vi "Abadines_Server3.vi"() -> ()   [LabVIEW 2013]
uses:
  <vilib>/NXT/Block Support/NXT_InputPort.ctl
  <vilib>/NXT/Block Support/NXT_MessageMailbox.ctl
  <vilib>/NXT/Block Support/NXT_OutputPort.ctl
  <vilib>/NXT/Subs/MotorOutput.ctl
  <vilib>/NXT/Dual Mode Library/BT/BlueTooth_Write_Num.vi
  <vilib>/NXT/NXTIO Xnodes/NXTIONodeSubVIs/NXTStopMotors.vi
  <vilib>/NXT/Dual Mode Library/Display/drawNumber.vi
  <vilib>/NXT/NXTIO Xnodes/AddressXNode/NXTIOAddress.xnode
  <vilib>/NXT/NXTIO Xnodes/NXTIOXNode/NXTIO.xnode
  <vilib>/NXT/Subs/LVHSConnector.ctl
  <vilib>/NXT/LegoClasses/BrickReference/BrickReference.lvclass
  <vilib>/NXT/Dual Mode Library/Display/drawNumber_float.vi
panel:
  out "Case Accord. BJr.":i32
  out "Blue Line":i16
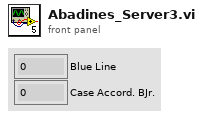
[diagram p1: front panel]
types:
  T1 = typedef "NXT_MessageMailbox.ctl" = u8
  T2 = typedef "LVHSConnector.ctl" = refnum<class "BrickReference.lvclass">
  T3 = typedef "NXT_OutputPort.ctl" = u8
  T4 = typedef "NXT_InputPort.ctl" = u32
  T5 = typedef "MotorOutput.ctl" = u8
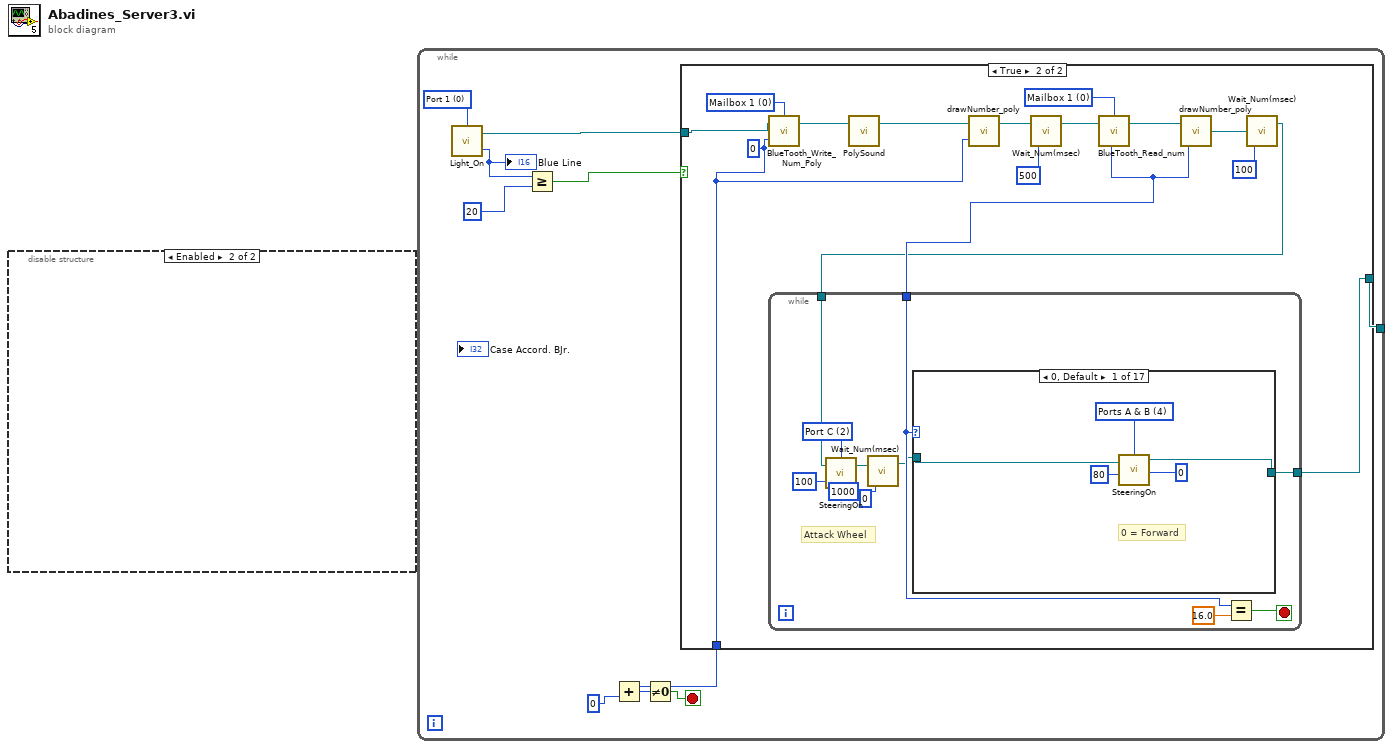
[diagram p0: block diagram]
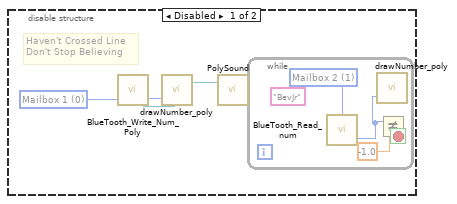
[diagram p2: hidden frame]
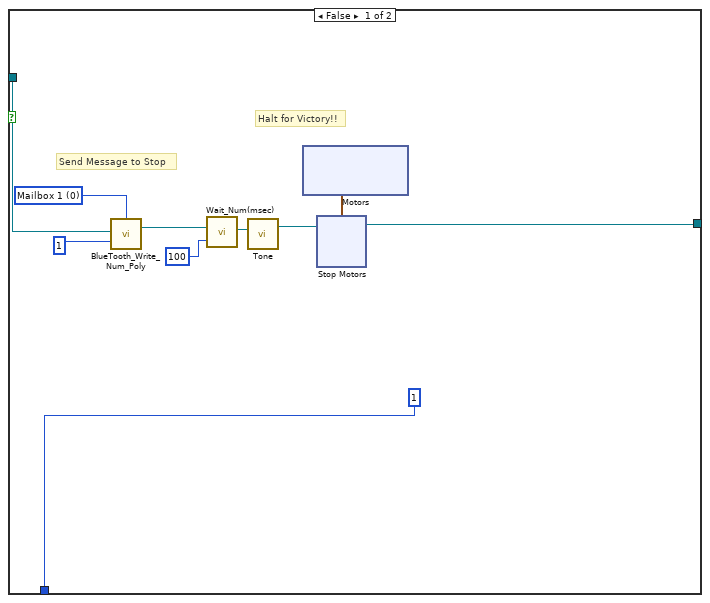
[diagram p3: hidden frame]
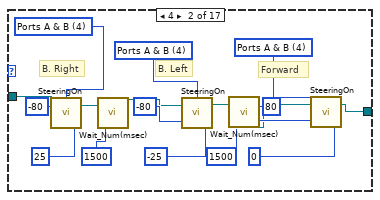
[diagram p4: hidden frame]
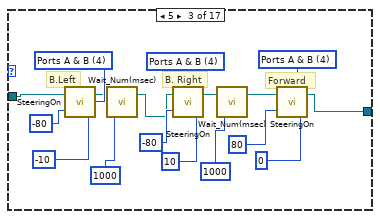
[diagram p5: hidden frame]
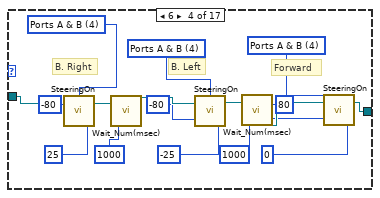
[diagram p6: hidden frame]
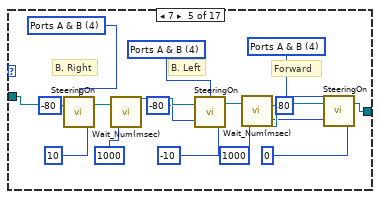
[diagram p7: hidden frame]
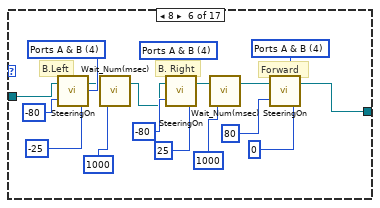
[diagram p8: hidden frame]
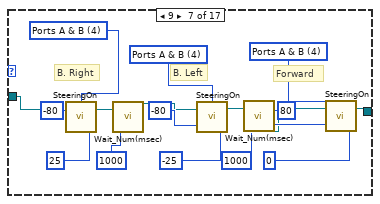
[diagram p9: hidden frame]
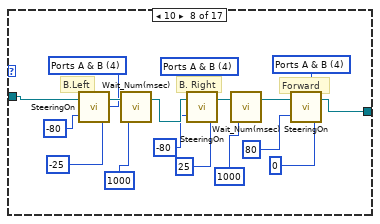
[diagram p10: hidden frame]
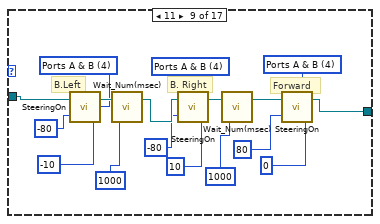
[diagram p11: hidden frame]
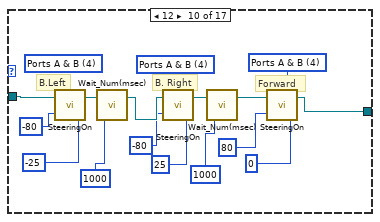
[diagram p12: hidden frame]
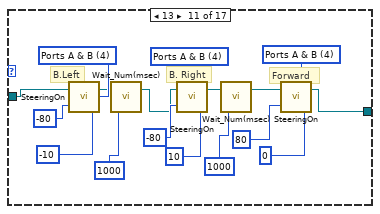
[diagram p13: hidden frame]
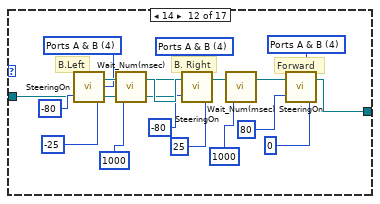
[diagram p14: hidden frame]
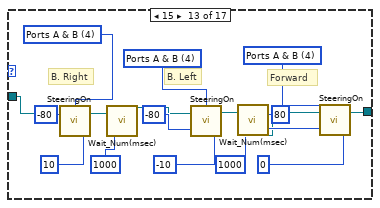
[diagram p15: hidden frame]
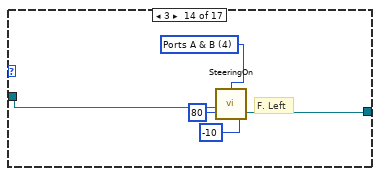
[diagram p16: hidden frame]
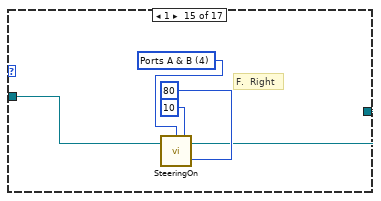
[diagram p17: hidden frame]
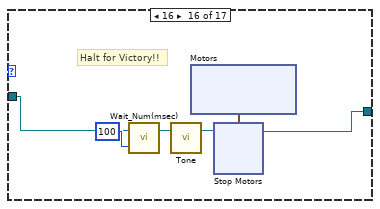
[diagram p18: hidden frame]
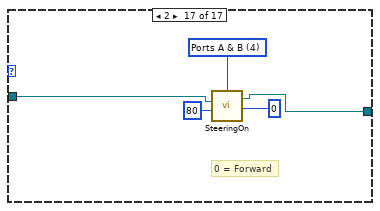
[diagram p19: hidden frame]
diagram:
  n1 = disable-structure shown="Enabled" {
    frame Disabled {
      w1 = T1 0 items=["Mailbox 1", "Mailbox 2", "Mailbox 3", "Mailbox 4", "Mailbox 5", "Mailbox 6", "Mailbox 7", "Mailbox 8", "Mailbox 9", "Mailbox 10"] ("Mailbox")
      # "Haven't Crossed Line\nDon't Stop Believing"
      n2 = call-poly <vilib>:"BlueTooth_Write_Num_Poly.vi"("Mailbox"=w1) -> ("Message"=w4:i32, 2:"NXT/EV3"=w2:T2, 4:"NXT/EV3"=w3:T2)  [unwired: 1 in]
      n3 = call-poly <vilib>:"drawNumber_poly.vi"("number"=w4, "NXT/EV3"=w3) -> ()  [unwired: 2 in, 1 out]
      n4 = call-poly <vilib>:"PolySound.vi"("NXT/EV3"=w3) -> ()  [unwired: 3 in, 1 out]
      n5 = while {
        stop <- _ stop-if-true
        w9 = T1 1 items=["Mailbox 1", "Mailbox 2", "Mailbox 3", "Mailbox 4", "Mailbox 5", "Mailbox 6", "Mailbox 7", "Mailbox 8", "Mailbox 9", "Mailbox 10"] ("Mailbox")
        (unwired) "BevJr" ("Partner Name")
        n6 = call <vilib>:"BlueTooth_Read_num.vi"("Mailbox"=w9) -> ("Message"=w5:i32, 2:"NXT/EV3"=w8:T2, 4:"NXT/EV3"=w7:T2)  [unwired: 1 in]
        n7 = call-poly <vilib>:"drawNumber_poly.vi"("number"=w5) -> ()  [unwired: 3 in, 1 out]
        n8 = Not Equal?(x=w5, y=-1.0) -> ()  [unwired: 1 out]
      }
    }
    frame Enabled {
    }
  }
  n9 = while {
    tunnel: [w15] -> _
    stop <- w11 stop-if-true
    w19 = T4 0 items=["Port 1", "Port 2", "Port 3", "Port 4"] ("Port (Port 3)")
    n10 = call <vilib>:"Light_On.vi"("Port (Port 3)"=w19) -> ("Scaled Value"=w18:i16, "NXT/EV3"=w10:T2)  [unwired: 2 in]
    "Blue Line" <- w18
    n11 = Greater Or Equal?(x=w18, y=i16 20) -> (x >= y?=w16:bool)
    n12 = case shown="True" w16 {
      tunnel: w10 -> [w27 w40]
      tunnel: [w21 w38] -> w15
      tunnel: [1 w39] -> w14
      frame False {
        w28 = T1 0 items=["Mailbox 1", "Mailbox 2", "Mailbox 3", "Mailbox 4", "Mailbox 5", "Mailbox 6", "Mailbox 7", "Mailbox 8", "Mailbox 9", "Mailbox 10"] ("Mailbox")
        # "Halt for Victory!!"
        # "Send Message to Stop"
        n13 = call-poly <vilib>:"BlueTooth_Write_Num_Poly.vi"("Message"=1, "NXT/EV3"=w27, "Mailbox"=w28) -> ("NXT/EV3"=w23:T2)  [unwired: 1 in]
        n14 = call <vilib>:"Wait_Num(msec).vi"("Time (100 msec)"=u32 100, "NXT/EV3"=w23) -> ("NXT/EV3"=w24:T2)  [unwired: 2 in]
        n15 = call <vilib>:"Tone.vi"("NXT/EV3"=w24) -> ("NXT/EV3"=w22:T2)  [unwired: 3 in]
        n16 = xnode "Motors"() -> ("Motor"=w20:cluster{"Port":T3, "Port":T3})
        n17 = xnode "Stop Motors"("Motors"=w20, "NXT/EV3"=w22) -> ("NXT/EV3"=w21:T2)
      }
      frame True {
        w50 = T1 0 items=["Mailbox 1", "Mailbox 2", "Mailbox 3", "Mailbox 4", "Mailbox 5", "Mailbox 6", "Mailbox 7", "Mailbox 8", "Mailbox 9", "Mailbox 10"] ("Mailbox")
        w39 = 0 ("Message")
        w41 = T1 0 items=["Mailbox 1", "Mailbox 2", "Mailbox 3", "Mailbox 4", "Mailbox 5", "Mailbox 6", "Mailbox 7", "Mailbox 8", "Mailbox 9", "Mailbox 10"] ("Mailbox")
        n18 = call-poly <vilib>:"BlueTooth_Write_Num_Poly.vi"("Message"=w39, "NXT/EV3"=w40, "Mailbox"=w41) -> ("NXT/EV3"=w42:T2)  [unwired: 1 in]
        n19 = call-poly <vilib>:"PolySound.vi"("NXT/EV3"=w42) -> ("NXT/EV3"=w47:T2)  [unwired: 3 in]
        n20 = call-poly <vilib>:"drawNumber_poly.vi"("number"=w39, "NXT/EV3"=w47) -> ("NXT/EV3"=w44:T2)  [unwired: 2 in]
        n21 = call <vilib>:"Wait_Num(msec).vi"("Time (100 msec)"=u32 500, "NXT/EV3"=w44) -> ("NXT/EV3"=w45:T2)  [unwired: 2 in]
        n22 = call <vilib>:"BlueTooth_Read_num.vi"("NXT/EV3"=w45, "Mailbox"=w50) -> ("Message"=w37:i32, "NXT/EV3"=w43:T2)  [unwired: 1 in]
        n23 = call-poly <vilib>:"drawNumber_poly.vi"("number"=w37, "NXT/EV3"=w43) -> ("NXT/EV3"=w49:T2)  [unwired: 2 in]
        n24 = call <vilib>:"Wait_Num(msec).vi"("Time (100 msec)"=u32 100, "NXT/EV3"=w49) -> ("NXT/EV3"=w36:T2)  [unwired: 2 in]
        n25 = while {
          tunnel: [w61] -> w38
          tunnel: w37 -> [w54]
          tunnel: w36 -> [w60]
          stop <- w56 stop-if-true
          w59 = T5 2 items=["Port A"=0, "Port B"=1, "Port C"=2, "Ports A & B"=4, "Ports A & C"=5, "Ports B & C"=6, "All Ports"=3] ("Output Ports (A & B)")
          # "Attack Wheel"
          n26 = call <vilib>:"SteeringOn.vi"("Power (75)"=100, "Steering (100)"=0, "NXT/EV3"=w60, "Output Ports (A & B)"=w59) -> ("NXT/EV3"=w53:T2)
          n27 = call <vilib>:"Wait_Num(msec).vi"("Time (100 msec)"=u32 1000, "NXT/EV3"=w53) -> ("NXT/EV3"=w52:T2)  [unwired: 2 in]
          n28 = case shown="0, Default" w54 {
            tunnel: w52 -> [w64 w77 w85 w102 w119 w145 w153 w170 w187 w204 w220 w237 w255 w272 w277 w282 w294]
            tunnel: [w63 w76 w84 w101 w118 w144 w152 w169 w186 w203 w219 w236 w254 w271 w276 w283 w293] -> w61
            frame 0, Default {
              w62 = T5 4 items=["Port A"=0, "Port B"=1, "Port C"=2, "Ports A & B"=4, "Ports A & C"=5, "Ports B & C"=6, "All Ports"=3] ("Output Ports (A & B) 5")
              # "0 = Forward"
              n29 = call <vilib>:"SteeringOn.vi"("Power (75)"=80, "Steering (100)"=0, "NXT/EV3"=w64, "Output Ports (A & B)"=w62) -> ("NXT/EV3"=w63:T2)
            }
            frame 4 {
              w73 = T5 4 items=["Port A"=0, "Port B"=1, "Port C"=2, "Ports A & B"=4, "Ports A & C"=5, "Ports B & C"=6, "All Ports"=3] ("Output Ports (A & B) 15")
              w74 = T5 4 items=["Port A"=0, "Port B"=1, "Port C"=2, "Ports A & B"=4, "Ports A & C"=5, "Ports B & C"=6, "All Ports"=3] ("Output Port (All Ports) 6")
              w75 = T5 4 items=["Port A"=0, "Port B"=1, "Port C"=2, "Ports A & B"=4, "Ports A & C"=5, "Ports B & C"=6, "All Ports"=3] ("Output Ports (A & B) 16")
              # "Forward"
              # "B. Left"
              # "B. Right"
              n30 = call <vilib>:"SteeringOn.vi"("Power (75)"=-80, "Steering (100)"=25, "NXT/EV3"=w77, "Output Ports (A & B)"=w75) -> ("NXT/EV3"=w72:T2)
              n31 = call <vilib>:"Wait_Num(msec).vi"("Time (100 msec)"=u32 1500, "NXT/EV3"=w72) -> ("NXT/EV3"=w71:T2)  [unwired: 2 in]
              n32 = call <vilib>:"SteeringOn.vi"("Power (75)"=-80, "Steering (100)"=-25, "NXT/EV3"=w71, "Output Ports (A & B)"=w74) -> ("NXT/EV3"=w70:T2)
              n33 = call <vilib>:"Wait_Num(msec).vi"("Time (100 msec)"=u32 1500, "NXT/EV3"=w70) -> ("NXT/EV3"=w69:T2)  [unwired: 2 in]
              n34 = call <vilib>:"SteeringOn.vi"("Power (75)"=80, "Steering (100)"=0, "NXT/EV3"=w69, "Output Ports (A & B)"=w73) -> ("NXT/EV3"=w76:T2)
            }
            frame 5 {
              w92 = T5 4 items=["Port A"=0, "Port B"=1, "Port C"=2, "Ports A & B"=4, "Ports A & C"=5, "Ports B & C"=6, "All Ports"=3] ("Output Ports (A & B) 21")
              w93 = T5 4 items=["Port A"=0, "Port B"=1, "Port C"=2, "Ports A & B"=4, "Ports A & C"=5, "Ports B & C"=6, "All Ports"=3] ("Output Port (All Ports) 9")
              w94 = T5 4 items=["Port A"=0, "Port B"=1, "Port C"=2, "Ports A & B"=4, "Ports A & C"=5, "Ports B & C"=6, "All Ports"=3] ("Output Ports (A & B) 22")
              # "Forward"
              # "B. Right"
              # "B.Left"
              n35 = call <vilib>:"SteeringOn.vi"("Power (75)"=-80, "Steering (100)"=-10, "NXT/EV3"=w85, "Output Ports (A & B)"=w94) -> ("NXT/EV3"=w90:T2)
              n36 = call <vilib>:"Wait_Num(msec).vi"("Time (100 msec)"=u32 1000, "NXT/EV3"=w90) -> ("NXT/EV3"=w89:T2)  [unwired: 2 in]
              n37 = call <vilib>:"SteeringOn.vi"("Power (75)"=-80, "Steering (100)"=10, "NXT/EV3"=w89, "Output Ports (A & B)"=w93) -> ("NXT/EV3"=w87:T2)
              n38 = call <vilib>:"Wait_Num(msec).vi"("Time (100 msec)"=u32 1000, "NXT/EV3"=w87) -> ("NXT/EV3"=w86:T2)  [unwired: 2 in]
              n39 = call <vilib>:"SteeringOn.vi"("Power (75)"=80, "Steering (100)"=0, "NXT/EV3"=w86, "Output Ports (A & B)"=w92) -> ("NXT/EV3"=w84:T2)
            }
            frame 6 {
              w111 = T5 4 items=["Port A"=0, "Port B"=1, "Port C"=2, "Ports A & B"=4, "Ports A & C"=5, "Ports B & C"=6, "All Ports"=3] ("Output Ports (A & B) 15")
              w110 = T5 4 items=["Port A"=0, "Port B"=1, "Port C"=2, "Ports A & B"=4, "Ports A & C"=5, "Ports B & C"=6, "All Ports"=3] ("Output Port (All Ports) 6")
              w109 = T5 4 items=["Port A"=0, "Port B"=1, "Port C"=2, "Ports A & B"=4, "Ports A & C"=5, "Ports B & C"=6, "All Ports"=3] ("Output Ports (A & B) 16")
              # "Forward"
              # "B. Left"
              # "B. Right"
              n40 = call <vilib>:"SteeringOn.vi"("Power (75)"=-80, "Steering (100)"=25, "NXT/EV3"=w102, "Output Ports (A & B)"=w109) -> ("NXT/EV3"=w112:T2)
              n41 = call <vilib>:"Wait_Num(msec).vi"("Time (100 msec)"=u32 1000, "NXT/EV3"=w112) -> ("NXT/EV3"=w113:T2)  [unwired: 2 in]
              n42 = call <vilib>:"SteeringOn.vi"("Power (75)"=-80, "Steering (100)"=-25, "NXT/EV3"=w113, "Output Ports (A & B)"=w110) -> ("NXT/EV3"=w114:T2)
              n43 = call <vilib>:"Wait_Num(msec).vi"("Time (100 msec)"=u32 1000, "NXT/EV3"=w114) -> ("NXT/EV3"=w115:T2)  [unwired: 2 in]
              n44 = call <vilib>:"SteeringOn.vi"("Power (75)"=80, "Steering (100)"=0, "NXT/EV3"=w115, "Output Ports (A & B)"=w111) -> ("NXT/EV3"=w101:T2)
            }
            frame 7 {
              w128 = T5 4 items=["Port A"=0, "Port B"=1, "Port C"=2, "Ports A & B"=4, "Ports A & C"=5, "Ports B & C"=6, "All Ports"=3] ("Output Ports (A & B) 15")
              w127 = T5 4 items=["Port A"=0, "Port B"=1, "Port C"=2, "Ports A & B"=4, "Ports A & C"=5, "Ports B & C"=6, "All Ports"=3] ("Output Port (All Ports) 6")
              w126 = T5 4 items=["Port A"=0, "Port B"=1, "Port C"=2, "Ports A & B"=4, "Ports A & C"=5, "Ports B & C"=6, "All Ports"=3] ("Output Ports (A & B) 16")
              # "Forward"
              # "B. Left"
              # "B. Right"
              n45 = call <vilib>:"SteeringOn.vi"("Power (75)"=-80, "Steering (100)"=10, "NXT/EV3"=w119, "Output Ports (A & B)"=w126) -> ("NXT/EV3"=w129:T2)
              n46 = call <vilib>:"Wait_Num(msec).vi"("Time (100 msec)"=u32 1000, "NXT/EV3"=w129) -> ("NXT/EV3"=w130:T2)  [unwired: 2 in]
              n47 = call <vilib>:"SteeringOn.vi"("Power (75)"=-80, "Steering (100)"=-10, "NXT/EV3"=w130, "Output Ports (A & B)"=w127) -> ("NXT/EV3"=w131:T2)
              n48 = call <vilib>:"Wait_Num(msec).vi"("Time (100 msec)"=u32 1000, "NXT/EV3"=w131) -> ("NXT/EV3"=w132:T2)  [unwired: 2 in]
              n49 = call <vilib>:"SteeringOn.vi"("Power (75)"=80, "Steering (100)"=0, "NXT/EV3"=w132, "Output Ports (A & B)"=w128) -> ("NXT/EV3"=w118:T2)
            }
            frame 8 {
              w141 = T5 4 items=["Port A"=0, "Port B"=1, "Port C"=2, "Ports A & B"=4, "Ports A & C"=5, "Ports B & C"=6, "All Ports"=3] ("Output Ports (A & B) 21")
              w142 = T5 4 items=["Port A"=0, "Port B"=1, "Port C"=2, "Ports A & B"=4, "Ports A & C"=5, "Ports B & C"=6, "All Ports"=3] ("Output Port (All Ports) 9")
              w143 = T5 4 items=["Port A"=0, "Port B"=1, "Port C"=2, "Ports A & B"=4, "Ports A & C"=5, "Ports B & C"=6, "All Ports"=3] ("Output Ports (A & B) 22")
              # "Forward"
              # "B. Right"
              # "B.Left"
              n50 = call <vilib>:"SteeringOn.vi"("Power (75)"=-80, "Steering (100)"=-25, "NXT/EV3"=w145, "Output Ports (A & B)"=w143) -> ("NXT/EV3"=w139:T2)
              n51 = call <vilib>:"Wait_Num(msec).vi"("Time (100 msec)"=u32 1000, "NXT/EV3"=w139) -> ("NXT/EV3"=w138:T2)  [unwired: 2 in]
              n52 = call <vilib>:"SteeringOn.vi"("Power (75)"=-80, "Steering (100)"=25, "NXT/EV3"=w138, "Output Ports (A & B)"=w142) -> ("NXT/EV3"=w136:T2)
              n53 = call <vilib>:"Wait_Num(msec).vi"("Time (100 msec)"=u32 1000, "NXT/EV3"=w136) -> ("NXT/EV3"=w135:T2)  [unwired: 2 in]
              n54 = call <vilib>:"SteeringOn.vi"("Power (75)"=80, "Steering (100)"=0, "NXT/EV3"=w135, "Output Ports (A & B)"=w141) -> ("NXT/EV3"=w144:T2)
            }
            frame 9 {
              w160 = T5 4 items=["Port A"=0, "Port B"=1, "Port C"=2, "Ports A & B"=4, "Ports A & C"=5, "Ports B & C"=6, "All Ports"=3] ("Output Ports (A & B) 15")
              w161 = T5 4 items=["Port A"=0, "Port B"=1, "Port C"=2, "Ports A & B"=4, "Ports A & C"=5, "Ports B & C"=6, "All Ports"=3] ("Output Port (All Ports) 6")
              w162 = T5 4 items=["Port A"=0, "Port B"=1, "Port C"=2, "Ports A & B"=4, "Ports A & C"=5, "Ports B & C"=6, "All Ports"=3] ("Output Ports (A & B) 16")
              # "Forward"
              # "B. Left"
              # "B. Right"
              n55 = call <vilib>:"SteeringOn.vi"("Power (75)"=-80, "Steering (100)"=25, "NXT/EV3"=w153, "Output Ports (A & B)"=w162) -> ("NXT/EV3"=w159:T2)
              n56 = call <vilib>:"Wait_Num(msec).vi"("Time (100 msec)"=u32 1000, "NXT/EV3"=w159) -> ("NXT/EV3"=w158:T2)  [unwired: 2 in]
              n57 = call <vilib>:"SteeringOn.vi"("Power (75)"=-80, "Steering (100)"=-25, "NXT/EV3"=w158, "Output Ports (A & B)"=w161) -> ("NXT/EV3"=w157:T2)
              n58 = call <vilib>:"Wait_Num(msec).vi"("Time (100 msec)"=u32 1000, "NXT/EV3"=w157) -> ("NXT/EV3"=w156:T2)  [unwired: 2 in]
              n59 = call <vilib>:"SteeringOn.vi"("Power (75)"=80, "Steering (100)"=0, "NXT/EV3"=w156, "Output Ports (A & B)"=w160) -> ("NXT/EV3"=w152:T2)
            }
            frame 10 {
              w179 = T5 4 items=["Port A"=0, "Port B"=1, "Port C"=2, "Ports A & B"=4, "Ports A & C"=5, "Ports B & C"=6, "All Ports"=3] ("Output Ports (A & B) 21")
              w178 = T5 4 items=["Port A"=0, "Port B"=1, "Port C"=2, "Ports A & B"=4, "Ports A & C"=5, "Ports B & C"=6, "All Ports"=3] ("Output Port (All Ports) 9")
              w177 = T5 4 items=["Port A"=0, "Port B"=1, "Port C"=2, "Ports A & B"=4, "Ports A & C"=5, "Ports B & C"=6, "All Ports"=3] ("Output Ports (A & B) 22")
              # "Forward"
              # "B. Right"
              # "B.Left"
              n60 = call <vilib>:"SteeringOn.vi"("Power (75)"=-80, "Steering (100)"=-25, "NXT/EV3"=w170, "Output Ports (A & B)"=w177) -> ("NXT/EV3"=w181:T2)
              n61 = call <vilib>:"Wait_Num(msec).vi"("Time (100 msec)"=u32 1000, "NXT/EV3"=w181) -> ("NXT/EV3"=w182:T2)  [unwired: 2 in]
              n62 = call <vilib>:"SteeringOn.vi"("Power (75)"=-80, "Steering (100)"=25, "NXT/EV3"=w182, "Output Ports (A & B)"=w178) -> ("NXT/EV3"=w184:T2)
              n63 = call <vilib>:"Wait_Num(msec).vi"("Time (100 msec)"=u32 1000, "NXT/EV3"=w184) -> ("NXT/EV3"=w185:T2)  [unwired: 2 in]
              n64 = call <vilib>:"SteeringOn.vi"("Power (75)"=80, "Steering (100)"=0, "NXT/EV3"=w185, "Output Ports (A & B)"=w179) -> ("NXT/EV3"=w169:T2)
            }
            frame 11 {
              w196 = T5 4 items=["Port A"=0, "Port B"=1, "Port C"=2, "Ports A & B"=4, "Ports A & C"=5, "Ports B & C"=6, "All Ports"=3] ("Output Ports (A & B) 21")
              w195 = T5 4 items=["Port A"=0, "Port B"=1, "Port C"=2, "Ports A & B"=4, "Ports A & C"=5, "Ports B & C"=6, "All Ports"=3] ("Output Port (All Ports) 9")
              w194 = T5 4 items=["Port A"=0, "Port B"=1, "Port C"=2, "Ports A & B"=4, "Ports A & C"=5, "Ports B & C"=6, "All Ports"=3] ("Output Ports (A & B) 22")
              # "Forward"
              # "B. Right"
              # "B.Left"
              n65 = call <vilib>:"SteeringOn.vi"("Power (75)"=-80, "Steering (100)"=-10, "NXT/EV3"=w187, "Output Ports (A & B)"=w194) -> ("NXT/EV3"=w198:T2)
              n66 = call <vilib>:"Wait_Num(msec).vi"("Time (100 msec)"=u32 1000, "NXT/EV3"=w198) -> ("NXT/EV3"=w199:T2)  [unwired: 2 in]
              n67 = call <vilib>:"SteeringOn.vi"("Power (75)"=-80, "Steering (100)"=10, "NXT/EV3"=w199, "Output Ports (A & B)"=w195) -> ("NXT/EV3"=w201:T2)
              n68 = call <vilib>:"Wait_Num(msec).vi"("Time (100 msec)"=u32 1000, "NXT/EV3"=w201) -> ("NXT/EV3"=w202:T2)  [unwired: 2 in]
              n69 = call <vilib>:"SteeringOn.vi"("Power (75)"=80, "Steering (100)"=0, "NXT/EV3"=w202, "Output Ports (A & B)"=w196) -> ("NXT/EV3"=w186:T2)
            }
            frame 12 {
              w212 = T5 4 items=["Port A"=0, "Port B"=1, "Port C"=2, "Ports A & B"=4, "Ports A & C"=5, "Ports B & C"=6, "All Ports"=3] ("Output Ports (A & B) 21")
              w211 = T5 4 items=["Port A"=0, "Port B"=1, "Port C"=2, "Ports A & B"=4, "Ports A & C"=5, "Ports B & C"=6, "All Ports"=3] ("Output Port (All Ports) 9")
              (unwired) T5 4 items=["Port A"=0, "Port B"=1, "Port C"=2, "Ports A & B"=4, "Ports A & C"=5, "Ports B & C"=6, "All Ports"=3] ("Output Ports (A & B) 22")
              # "Forward"
              # "B. Right"
              # "B.Left"
              n70 = call <vilib>:"SteeringOn.vi"("Power (75)"=-80, "Steering (100)"=-25, "NXT/EV3"=w204) -> ("NXT/EV3"=w214:T2)  [unwired: 1 in]
              n71 = call <vilib>:"Wait_Num(msec).vi"("Time (100 msec)"=u32 1000, "NXT/EV3"=w214) -> ("NXT/EV3"=w215:T2)  [unwired: 2 in]
              n72 = call <vilib>:"SteeringOn.vi"("Power (75)"=-80, "Steering (100)"=25, "NXT/EV3"=w215, "Output Ports (A & B)"=w211) -> ("NXT/EV3"=w217:T2)
              n73 = call <vilib>:"Wait_Num(msec).vi"("Time (100 msec)"=u32 1000, "NXT/EV3"=w217) -> ("NXT/EV3"=w218:T2)  [unwired: 2 in]
              n74 = call <vilib>:"SteeringOn.vi"("Power (75)"=80, "Steering (100)"=0, "NXT/EV3"=w218, "Output Ports (A & B)"=w212) -> ("NXT/EV3"=w203:T2)
            }
            frame 13 {
              w227 = T5 4 items=["Port A"=0, "Port B"=1, "Port C"=2, "Ports A & B"=4, "Ports A & C"=5, "Ports B & C"=6, "All Ports"=3] ("Output Ports (A & B) 21")
              w228 = T5 4 items=["Port A"=0, "Port B"=1, "Port C"=2, "Ports A & B"=4, "Ports A & C"=5, "Ports B & C"=6, "All Ports"=3] ("Output Port (All Ports) 9")
              w229 = T5 4 items=["Port A"=0, "Port B"=1, "Port C"=2, "Ports A & B"=4, "Ports A & C"=5, "Ports B & C"=6, "All Ports"=3] ("Output Ports (A & B) 22")
              # "Forward"
              # "B. Right"
              # "B.Left"
              n75 = call <vilib>:"SteeringOn.vi"("Power (75)"=-80, "Steering (100)"=-10, "NXT/EV3"=w220, "Output Ports (A & B)"=w229) -> ("NXT/EV3"=w225:T2)
              n76 = call <vilib>:"Wait_Num(msec).vi"("Time (100 msec)"=u32 1000, "NXT/EV3"=w225) -> ("NXT/EV3"=w224:T2)  [unwired: 2 in]
              n77 = call <vilib>:"SteeringOn.vi"("Power (75)"=-80, "Steering (100)"=10, "NXT/EV3"=w224, "Output Ports (A & B)"=w228) -> ("NXT/EV3"=w222:T2)
              n78 = call <vilib>:"Wait_Num(msec).vi"("Time (100 msec)"=u32 1000, "NXT/EV3"=w222) -> ("NXT/EV3"=w221:T2)  [unwired: 2 in]
              n79 = call <vilib>:"SteeringOn.vi"("Power (75)"=80, "Steering (100)"=0, "NXT/EV3"=w221, "Output Ports (A & B)"=w227) -> ("NXT/EV3"=w219:T2)
            }
            frame 14 {
              w246 = T5 4 items=["Port A"=0, "Port B"=1, "Port C"=2, "Ports A & B"=4, "Ports A & C"=5, "Ports B & C"=6, "All Ports"=3] ("Output Ports (A & B) 21")
              w245 = T5 4 items=["Port A"=0, "Port B"=1, "Port C"=2, "Ports A & B"=4, "Ports A & C"=5, "Ports B & C"=6, "All Ports"=3] ("Output Port (All Ports) 9")
              w244 = T5 4 items=["Port A"=0, "Port B"=1, "Port C"=2, "Ports A & B"=4, "Ports A & C"=5, "Ports B & C"=6, "All Ports"=3] ("Output Ports (A & B) 22")
              # "Forward"
              # "B. Right"
              # "B.Left"
              n80 = call <vilib>:"SteeringOn.vi"("Power (75)"=-80, "Steering (100)"=-25, "NXT/EV3"=w237, "Output Ports (A & B)"=w244) -> ("NXT/EV3"=w248:T2)
              n81 = call <vilib>:"Wait_Num(msec).vi"("Time (100 msec)"=u32 1000, "NXT/EV3"=w248) -> ("NXT/EV3"=w249:T2)  [unwired: 2 in]
              n82 = call <vilib>:"SteeringOn.vi"("Power (75)"=-80, "Steering (100)"=25, "NXT/EV3"=w249, "Output Ports (A & B)"=w245) -> ("NXT/EV3"=w251:T2)
              n83 = call <vilib>:"Wait_Num(msec).vi"("Time (100 msec)"=u32 1000, "NXT/EV3"=w251) -> ("NXT/EV3"=w252:T2)  [unwired: 2 in]
              n84 = call <vilib>:"SteeringOn.vi"("Power (75)"=80, "Steering (100)"=0, "NXT/EV3"=w252, "Output Ports (A & B)"=w246) -> ("NXT/EV3"=w236:T2)
            }
            frame 15 {
              w262 = T5 4 items=["Port A"=0, "Port B"=1, "Port C"=2, "Ports A & B"=4, "Ports A & C"=5, "Ports B & C"=6, "All Ports"=3] ("Output Ports (A & B) 15")
              w263 = T5 4 items=["Port A"=0, "Port B"=1, "Port C"=2, "Ports A & B"=4, "Ports A & C"=5, "Ports B & C"=6, "All Ports"=3] ("Output Port (All Ports) 6")
              w253 = T5 4 items=["Port A"=0, "Port B"=1, "Port C"=2, "Ports A & B"=4, "Ports A & C"=5, "Ports B & C"=6, "All Ports"=3] ("Output Ports (A & B) 16")
              # "Forward"
              # "B. Left"
              # "B. Right"
              n85 = call <vilib>:"SteeringOn.vi"("Power (75)"=-80, "Steering (100)"=10, "NXT/EV3"=w255, "Output Ports (A & B)"=w253) -> ("NXT/EV3"=w261:T2)
              n86 = call <vilib>:"Wait_Num(msec).vi"("Time (100 msec)"=u32 1000, "NXT/EV3"=w261) -> ("NXT/EV3"=w260:T2)  [unwired: 2 in]
              n87 = call <vilib>:"SteeringOn.vi"("Power (75)"=-80, "Steering (100)"=-10, "NXT/EV3"=w260, "Output Ports (A & B)"=w263) -> ("NXT/EV3"=w259:T2)
              n88 = call <vilib>:"Wait_Num(msec).vi"("Time (100 msec)"=u32 1000, "NXT/EV3"=w259) -> ("NXT/EV3"=w258:T2)  [unwired: 2 in]
              n89 = call <vilib>:"SteeringOn.vi"("Power (75)"=80, "Steering (100)"=0, "NXT/EV3"=w258, "Output Ports (A & B)"=w262) -> ("NXT/EV3"=w254:T2)
            }
            frame 3 {
              w270 = T5 4 items=["Port A"=0, "Port B"=1, "Port C"=2, "Ports A & B"=4, "Ports A & C"=5, "Ports B & C"=6, "All Ports"=3] ("Output Port (All Ports) 3")
              # "F. Left"
              n90 = call <vilib>:"SteeringOn.vi"("Power (75)"=80, "Steering (100)"=-10, "NXT/EV3"=w272, "Output Ports (A & B)"=w270) -> ("NXT/EV3"=w271:T2)
            }
            frame 1 {
              w275 = T5 4 items=["Port A"=0, "Port B"=1, "Port C"=2, "Ports A & B"=4, "Ports A & C"=5, "Ports B & C"=6, "All Ports"=3] ("Output Ports (A & B) 12")
              # "F.  Right"
              n91 = call <vilib>:"SteeringOn.vi"("Power (75)"=80, "Steering (100)"=10, "NXT/EV3"=w277, "Output Ports (A & B)"=w275) -> ("NXT/EV3"=w276:T2)
            }
            frame 16 {
              # "Halt for Victory!!"
              n92 = call <vilib>:"Wait_Num(msec).vi"("Time (100 msec)"=u32 100, "NXT/EV3"=w282) -> ("NXT/EV3"=w281:T2)  [unwired: 2 in]
              n93 = call <vilib>:"Tone.vi"("NXT/EV3"=w281) -> ("NXT/EV3"=w280:T2)  [unwired: 3 in]
              n94 = xnode "Motors"() -> ("Motor"=w285:cluster{"Port":T3, "Port":T3})
              n95 = xnode "Stop Motors"("Motors"=w285, "NXT/EV3"=w280) -> ("NXT/EV3"=w283:T2)
            }
            frame 2 {
              w292 = T5 4 items=["Port A"=0, "Port B"=1, "Port C"=2, "Ports A & B"=4, "Ports A & C"=5, "Ports B & C"=6, "All Ports"=3] ("Output Ports (A & B) 10")
              # "0 = Forward"
              n96 = call <vilib>:"SteeringOn.vi"("Power (75)"=80, "Steering (100)"=0, "NXT/EV3"=w294, "Output Ports (A & B)"=w292) -> ("NXT/EV3"=w293:T2)
            }
          }
          n97 = Equal?(x=w54, y=16.0) -> (x = y?=w56:bool)
        }
      }
    }
    n98 = Add(x=w14, y=0) -> (x+y=w12:i32)
    n99 = Not Equal To 0?(x=w12) -> (x != 0?=w11:bool)
  }
